vi "Device_manage.vi"() -> ()   [LabVIEW 2010]
uses:
  libdaqVI.lvlib
panel:
  out "采集卡状态":bool
  in  "操作函数类型选择":enum32{"byindex ", "byname"}(radio)
  in  "UID指示灯":bool
  in  "rename":bool
  in  "设备新名称":string
  in  "退出程序":bool
  out "设备名称":string
  out "设备数量":u32
  # "设备管理演示程序"
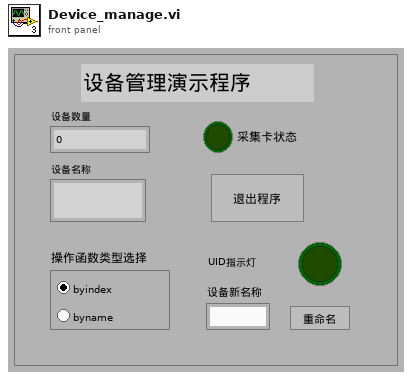
[diagram p1: front panel]
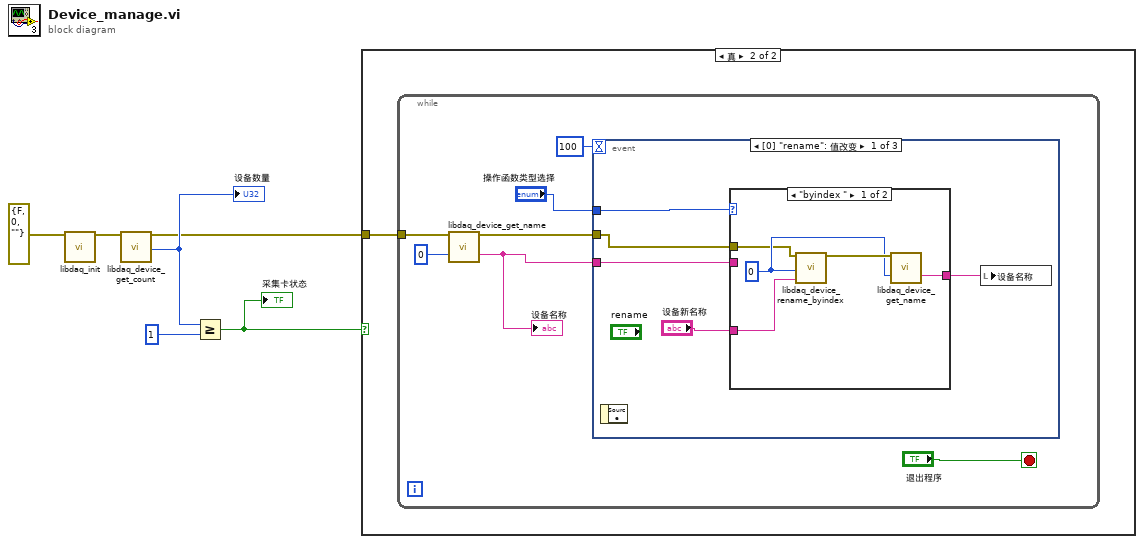
[diagram p0: block diagram]
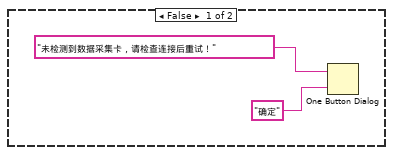
[diagram p2: hidden frame]
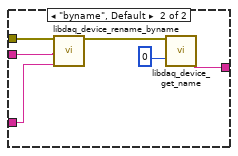
[diagram p3: hidden frame]
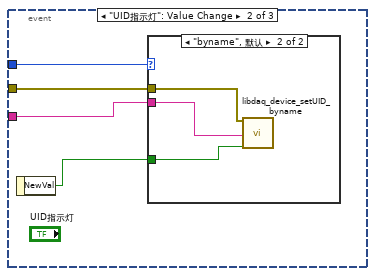
[diagram p4: hidden frame]
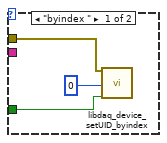
[diagram p5: hidden frame]
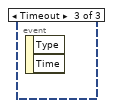
[diagram p6: hidden frame]
diagram:
  n1 = call "libdaq_init.vi"("error in (no error)"=errorcluster {"status"=FALSE, "code"=0, "source"=""}) -> ("error out"=w6:errorcluster)  [unwired: 18 in]
  n2 = call "libdaq_device_get_count.vi"("error in (no error)"=w6) -> ("error out"=w1:errorcluster, "device_count"=w2:i32)  [unwired: 17 in]
  "设备数量" <- w2
  n3 = Greater Or Equal?(x=w2, y=u32 1 ("name length")) -> (x >= y?=w3:bool)
  "采集卡状态" <- w3
  n4 = case shown="真" w3 {
    tunnel: w1 -> [_ w9]
    frame False {
      n5 = One Button Dialog(message="未检测到数据采集卡，请检查连接后重试！" ("消息"), button name ("OK")="确定" ("按钮名称（“确定”）")) -> ()  [unwired: 1 out]
    }
    frame True {
      n6 = while {
        tunnel: w9 -> [w13]
        stop <- "退出程序" stop-if-true
        n7 = call "libdaq_device_get_name.vi"("error in (no error)"=w13, "device_index"=u32 0 ("name length")) -> ("error out"=w11:errorcluster, "device_name"=w10:string)  [unwired: 16 in]
        "设备名称" <- w10
        n8 = event shown="[0] \"rename\": 值改变" {
          selector: _ -> [_ _ _]
          dyn-events: _ -> [_ _ _]
          timeout: 100 -> [_ _ _]
          tunnel: "操作函数类型选择" -> [w21 w35 _]
          tunnel: w10 -> [w20 w34 _]
          tunnel: w11 -> [w17 w33 _]
          event "rename": Value Change {
            n9 = event-data() -> ()  [unwired: 1 in, 1 out]
            n10 = case shown="\"byindex \"" w21 {
              tunnel: w20 -> [_ w29]
              tunnel: "设备新名称" -> [w25 w27]
              tunnel: [w23 w31] -> w18
              tunnel: w17 -> [w22 w28]
              frame "byindex " {
                w24 = u32 0 ("name length")
                n11 = call "libdaq_device_rename_byindex.vi"("error in (no error)"=w22, "device_index"=w24, "newname"=w25) -> ("error out"=w26:errorcluster)  [unwired: 16 in]
                n12 = call "libdaq_device_get_name.vi"("error in (no error)"=w26, "device_index"=w24) -> ("device_name"=w23:string)  [unwired: 16 in, 1 out]
              }
              frame "byname", Default {
                n13 = call "libdaq_device_rename_byname.vi"("error in (no error)"=w28, "device_name"=w29, "newname"=w27) -> ("error out"=w30:errorcluster)  [unwired: 16 in]
                n14 = call "libdaq_device_get_name.vi"("error in (no error)"=w30, "device_index"=u32 0 ("name length")) -> ("device_name"=w31:string)  [unwired: 16 in, 1 out]
              }
            }
            n15 = local write "设备名称"(w18) -> ()
          }
          event "UID指示灯": Value Change {
            n16 = event-data() -> ("NewVal"=w36:bool)  [unwired: 1 in]
            n17 = case shown="\"byname\", 默认" w35 {
              tunnel: w36 -> [w39 w42]
              tunnel: w34 -> [_ w41]
              tunnel: w33 -> [w37 w40]
              frame "byindex " {
                n18 = call "libdaq_device_setUID_byindex.vi"("error in (no error)"=w37, "device_index"=u32 0 ("name length"), "UID state"=w39) -> ()  [unwired: 16 in, 1 out]
              }
              frame "byname", Default {
                n19 = call "libdaq_device_setUID_byname.vi"("error in (no error)"=w40, "device_name"=w41, "UID state"=w42) -> ()  [unwired: 16 in, 1 out]
              }
            }
          }
          event Timeout {
            n20 = event-data() -> ()  [unwired: 1 in, 2 out]
          }
        }
      }
    }
  }
